vi "JSON command parser.vi"(11 "JSON command":string) -> (0 "Value":dbl, 3 "Command string":string)   [LabVIEW 2014]
uses:
  <vilib>/addons/JSON API/JSON Value/Set from JSON string.vi
  <vilib>/addons/JSON API/JSON Scalar/Get as Text.vi
  <vilib>/addons/JSON API/JSON Scalar/Get as DBL.vi
  <vilib>/addons/JSON API/JSON Value/JSON Value.lvclass
  <vilib>/addons/JSON API/Get Polymorphic/JSON GetSet.lvlib
  <vilib>/addons/JSON API/JSON Scalar/JSON Scalar.lvclass
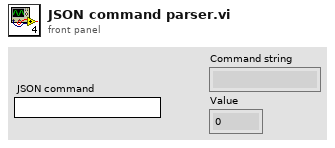
[diagram p1: front panel]
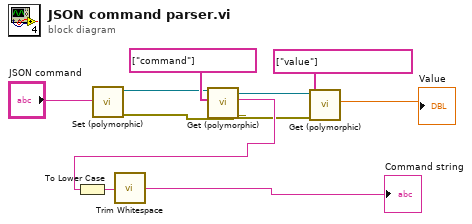
[diagram p0: block diagram]
diagram:
  n1 = call-poly <vilib>:"Set (polymorphic).vi"("JSON stream"="JSON command") -> ("error out"=w5:errorcluster, "JSON Value out"=w4:refnum<class "JSON Value.lvclass">)  [unwired: 8 in, 1 out]
  n2 = call-poly <vilib>:"Get (polymorphic).vi"("error in (no error)"=w5, "Name Array"=string[] ["command"], "JSON Scalar in"=w4) -> ("error out"=w7:errorcluster, "LabVIEW Text"=w10:string, "JSON Scalar out"=w8:refnum<class "JSON Value.lvclass">)  [unwired: 6 in]
  n3 = To Lower Case(string=w10) -> (all lower case string=w11:string)
  n4 = call <vilib>:"Trim Whitespace.vi"("string"=w11) -> ("trimmed string"=→"Command string":string)  [unwired: 1 in]
  n5 = call-poly <vilib>:"Get (polymorphic).vi"("error in (no error)"=w7, "Name Array"=string[] ["value"], "JSON Value in"=w8) -> ("Number"=→"Value":dbl)  [unwired: 6 in, 2 out]
